vi "MessageName.vi"() -> (2 "MessageName":string)   [LabVIEW 2020, in "UdpPayload.lvlib"]
uses:
  UdpPayload.lvlib
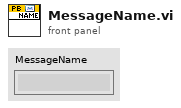
[diagram p1: front panel]
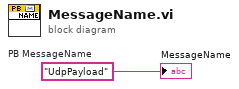
[diagram p0: block diagram]
diagram:
  w1 = "UdpPayload"  # PB MessageName
  "MessageName" <- w1
